vi "Read Cancel build.vi"(11 "BuildManager in":refnum<class "BuildManager.lvclass">) -> (2 "Cancel?":bool, 3 "BuildManager out":refnum<class "BuildManager.lvclass">)   [LabVIEW 2019, in "SolutionBuilder.lvlib" / "BuildManager.lvclass"]
uses:
  BuildManager.lvclass
  BuildManager.lvclass/BuildManager.ctl
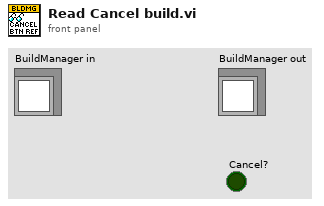
[diagram p1: front panel]
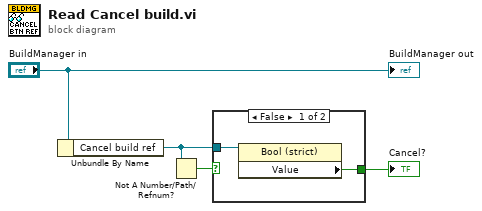
[diagram p0: block diagram]
diagram:
  n1 = Unbundle By Name("BuildManager in") -> ("Cancel build ref"=w2:refnum<vi>)
  n2 = Not A Number/Path/Refnum?(number/path/refnum=w2) -> (NaN/Path/Refnum?=w1:bool)
  n3 = case shown="False" w1 {
    tunnel: [w6 _] -> w3
    tunnel: w2 -> [w5 _]
    frame False {
      n4 = property class="Bool (strict)"(reference=w5) -> ("Value"=w6:bool)  [unwired: 1 in, 2 out]
    }
    frame True {
    }
  }
  "Cancel?" <- w3
  "BuildManager out" <- "BuildManager in"
